vi "PumpControl_final.vi"() -> ()   [LabVIEW 2017]
uses:
  <vilib>/Utility/error.llb/Error Cluster From Error Code.vi
  <vilib>/ErrorRing/Error Ring.xnode
panel:
  out "PUMP OFF":bool
  out "PUMP ON":bool
  out "Tank":dbl(slide) scale=0.0..10.0
  in  "Stop pump at:":dbl=3.0
  in  "Start pump over:":dbl=6.0
  in  "stop":bool
  # "PUMP CONTROL"
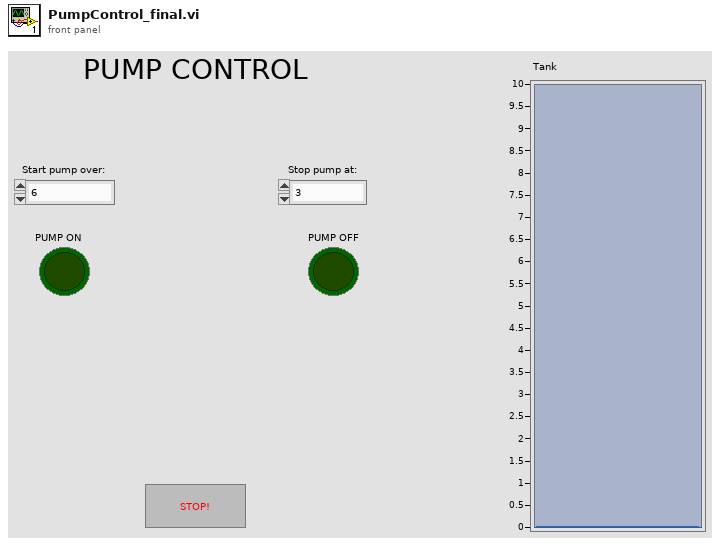
[diagram p1: front panel]
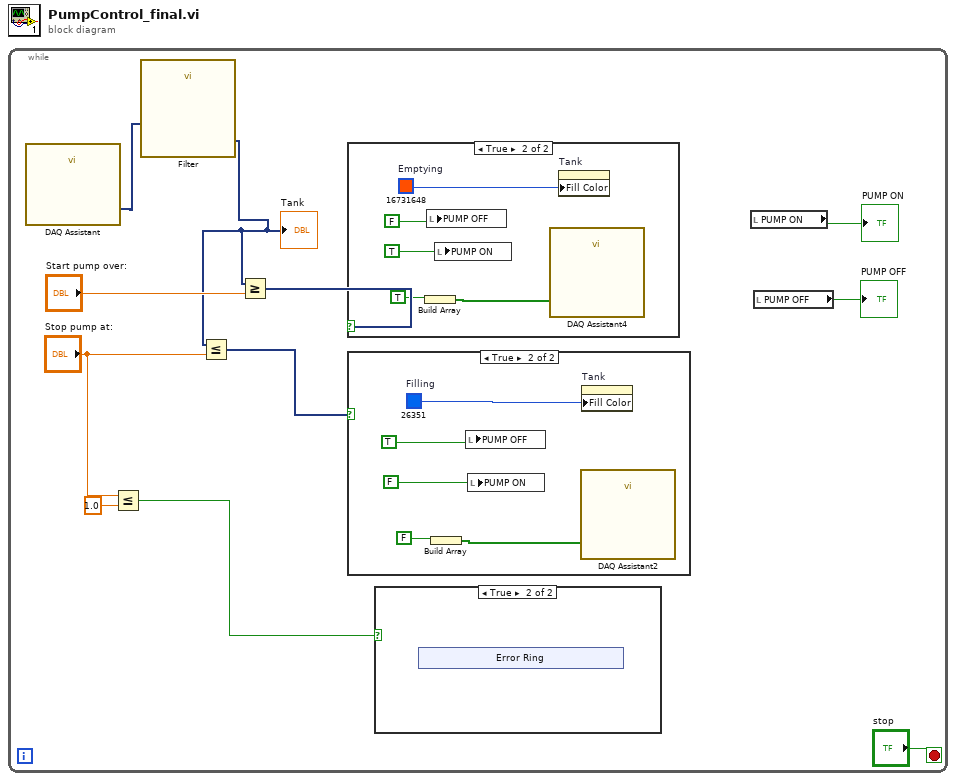
[diagram p0: block diagram]
diagram:
  n1 = while {
    stop <- "stop" stop-if-true
    n2 = call "DAQ Assistant"() -> ("data"=w2:dynamicdata)  [unwired: 17 in, 2 out]
    n3 = Less Or Equal?(x="Stop pump at:", y=1.0) -> (x <= y?=w5:bool)
    n4 = call "Filter"("Signal"=w2) -> ("Filtered Signal"=w1:dynamicdata)  [unwired: 9 in, 1 out]
    "Tank" <- w1
    n5 = Less Or Equal?(x=w1, y="Stop pump at:") -> (x <= y?=w8:dynamicdata)
    n6 = Greater Or Equal?(x=w1, y="Start pump over:") -> (x >= y?=w9:dynamicdata)
    n7 = case shown="True" w9 {
      frame False {
      }
      frame True {
        w22 = u32 16731648  # Emptying
        n8 = Build Array(TRUE) -> (w25:bool[])
        n9 = local write "PUMP OFF"(FALSE) -> ()
        n10 = local write "PUMP ON"(TRUE) -> ()
        n11 = call "DAQ Assistant4"("data"=w25) -> ()  [unwired: 17 in, 2 out]
        n12 = property on="Tank" class="Slide (strict)"("Fill Color"=w22) -> ()  [unwired: 2 in, 2 out]
      }
    }
    n13 = case shown="True" w8 {
      frame False {
      }
      frame True {
        w17 = u32 26351  # Filling
        n14 = Build Array(FALSE) -> (w20:bool[])
        n15 = local write "PUMP OFF"(TRUE) -> ()
        n16 = local write "PUMP ON"(FALSE) -> ()
        n17 = call "DAQ Assistant2"("data"=w20) -> ()  [unwired: 17 in, 2 out]
        n18 = property on="Tank" class="Slide (strict)"("Fill Color"=w17) -> ()  [unwired: 2 in, 2 out]
      }
    }
    n19 = case shown="True" w5 {
      frame False {
      }
      frame True {
        n20 = xnode ("Error Ring")() -> ()  [unwired: 1 out]
      }
    }
    n21 = local read "PUMP ON"() -> (→"PUMP ON":bool)
    n22 = local read "PUMP OFF"() -> (→"PUMP OFF":bool)
  }
